vi "UIRef.vi"(8 "error in":errorcluster, 11 "node in":refnum<class "LabVIEW Build Node.lvclass">) -> (0 "error out":errorcluster, 2 "VI refnum":refnum<vi>, 3 "node out":refnum<class "LabVIEW Build Node.lvclass">)   [LabVIEW 2014, in "LabVIEW Build Node.lvclass"]
doc: "Stores the static reference to the UI of the node."
uses:
  LabVIEW Build Node.lvclass
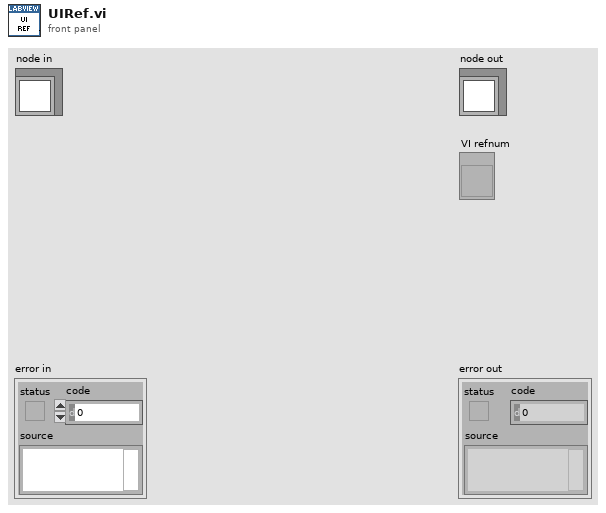
[diagram p1: front panel]
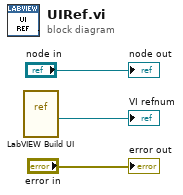
[diagram p0: block diagram]
diagram:
  n1 = vi-ref "LabVIEW Build UI.vi"() -> (→"VI refnum":refnum<vi>)
  "error out" <- "error in"
  "node out" <- "node in"
